vi "uc480_PixelPeek.vi"() -> ()   [LabVIEW 2011]
uses:
  C:/Program Files/Thorlabs/Scientific Imaging/DCx Camera Support/Develop/DotNet/uc480DotNet.dll
  Develop/DotNet/uc480DotNet.dll
panel:
  out "Maus":T1
  out "Blue":i32
  out "Green":i32
  out "Red":i32
  out "X":i32
  out "Y":i32
  out "Image":picture
  in  "Camera ID":i32 min=0 max=255
  out "Serial Number":string
  out "AOI Height":i32=8
  out "AOI Width":i32=8
  out "Bits/Pixel":i32=8
  out "Error Out":errorcluster caption="error"
  in  "Exit Camera":bool
  in  "Init Camera":bool
  # "Coordinates"
  # "Pixel Values"
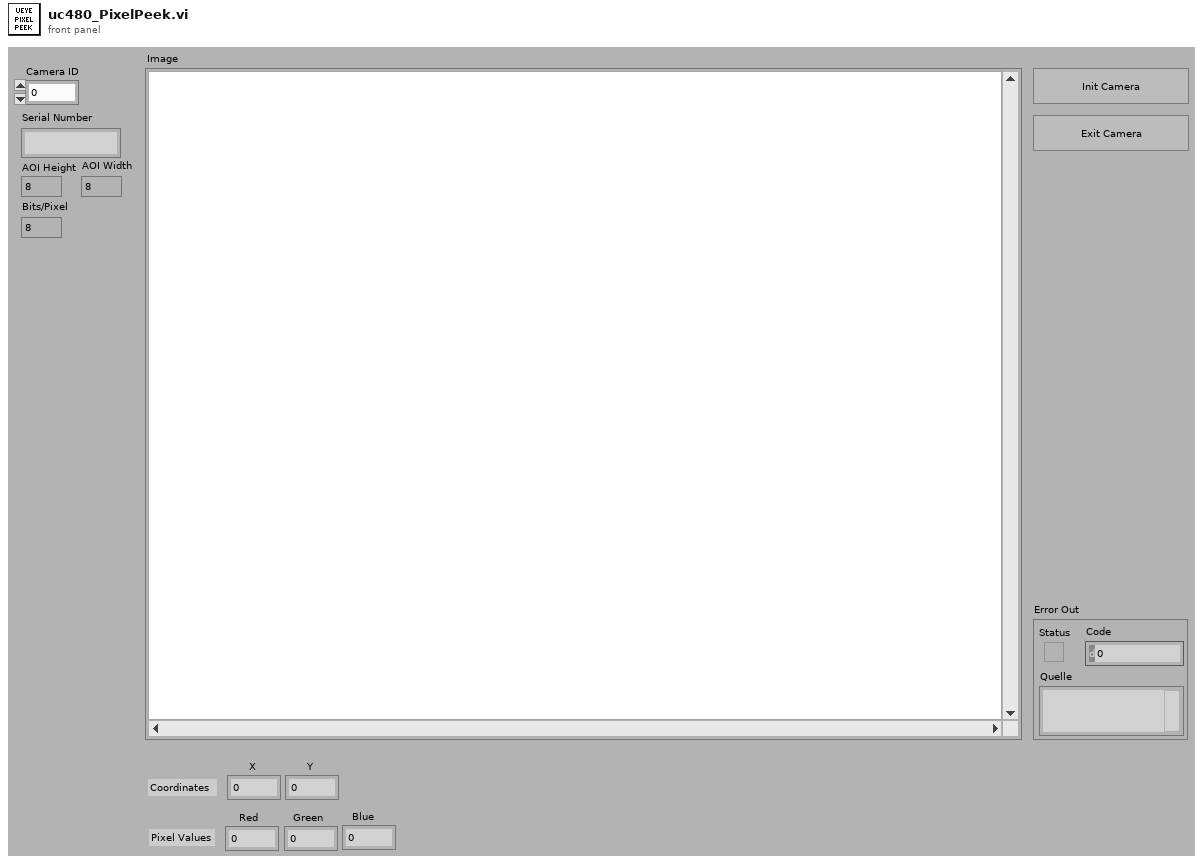
[diagram p1: front panel]
types:
  T1 = cluster{"Mouse Position":cluster{"X":i32, "Y":i32}, "Mouse Modifiers":cluster{"Button Down":bool, "Shift Mod":bool, "Menu Mod":bool, "Option Mod":bool}}
  T2 = enum8{"Enabled", "Disabled", "Disabled and Grayed Out"}
  T3 = typedef "LVMouseTypeDef.ctl" = cluster{"Mouse Position":cluster{"X":i32, "Y":i32}, "Mouse Modifiers":cluster{"Button Down":bool, "Shift Mod":bool, "Menu Mod":bool, "Option Mod":bool}}
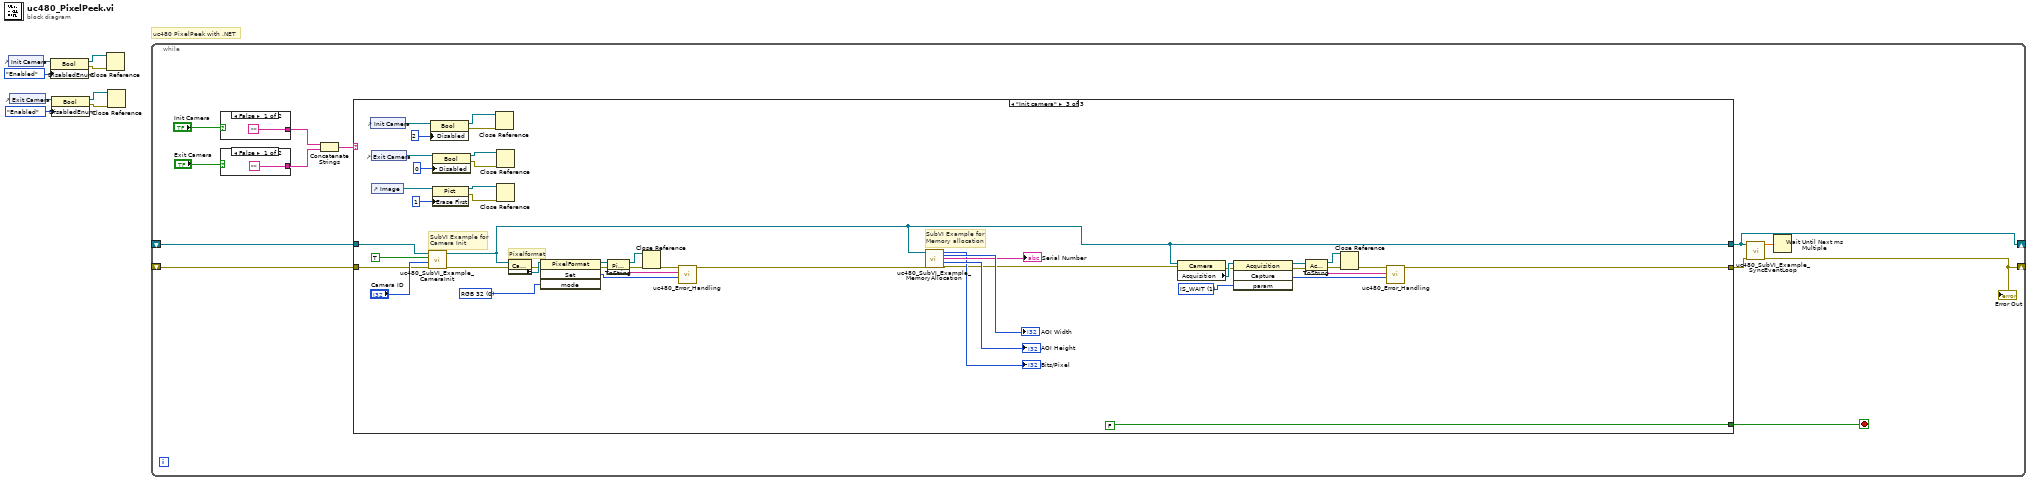
[diagram p0: block diagram]
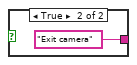
[diagram p2: hidden frame]
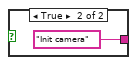
[diagram p3: hidden frame]
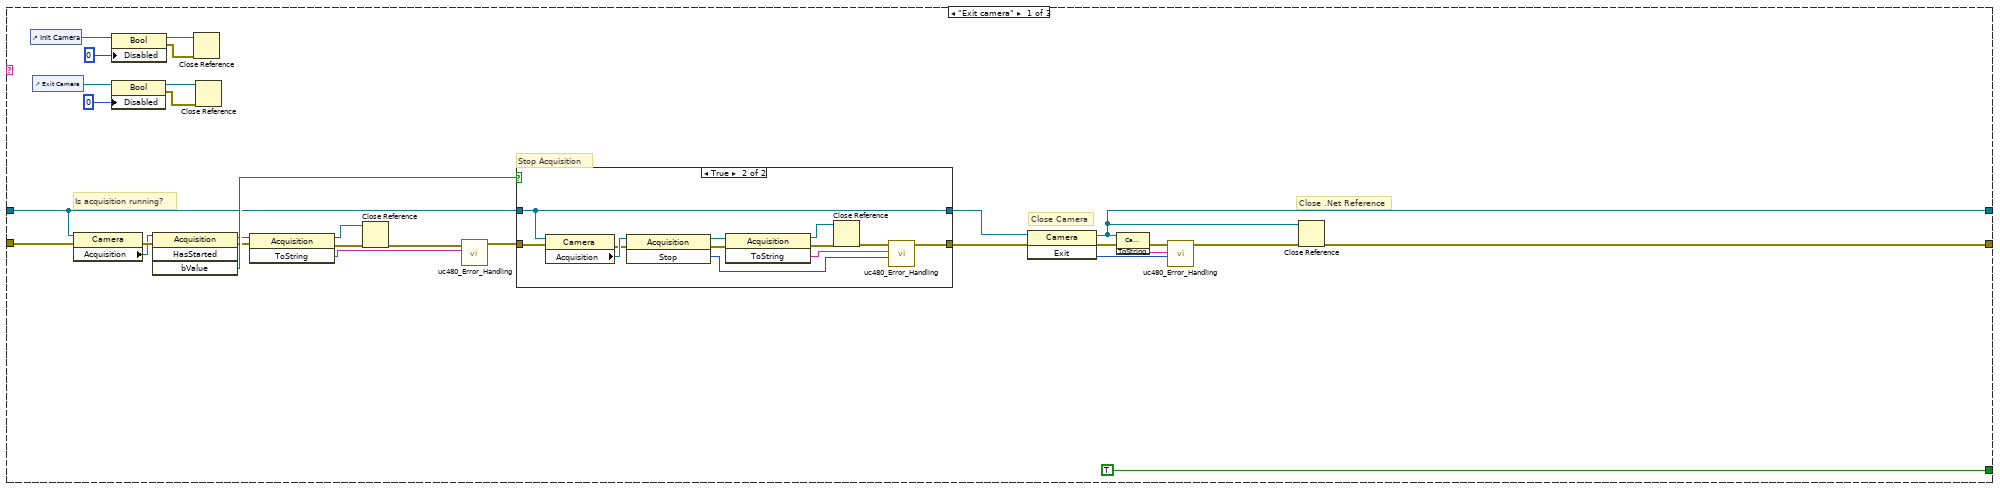
[diagram p4: hidden frame]
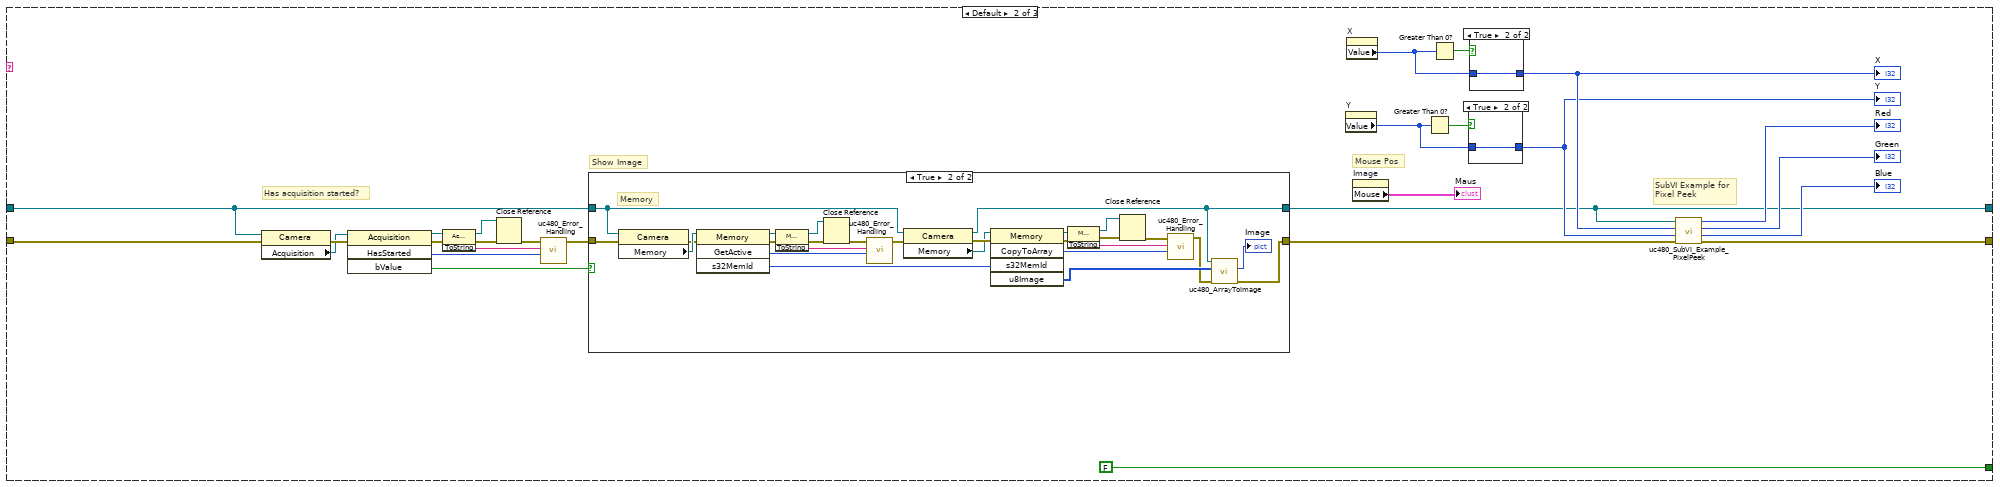
[diagram p6: hidden frame]
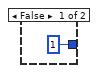
[diagram p7: hidden frame]
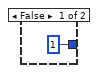
[diagram p8: hidden frame]
diagram:
  # "uc480 PixelPeek with .NET"
  n1 = control-ref of="Init Camera"() -> (w7:refnum<vi>)
  n2 = control-ref of="Exit Camera"() -> (w5:refnum<vi>)
  n3 = property class="Bool"(reference=w7, "DisabledEnum"=T2."Enabled" ("Disabled")) -> (reference out=w3:refnum<vi>, error out=w4:errorcluster)  [unwired: 1 in]
  n4 = property class="Bool"(reference=w5, "DisabledEnum"=T2."Enabled" ("Disabled")) -> (reference out=w2:refnum<vi>, error out=w1:errorcluster)  [unwired: 1 in]
  n5 = Close Reference ("Close Referenz")(reference=w3, error in (no error)=w4) -> ()  [unwired: 1 out]
  n6 = Close Reference ("Close Referenz")(reference=w2, error in (no error)=w1) -> ()  [unwired: 1 out]
  n7 = while {
    shift-right: [w12] -> _
    shift-left: _ -> [w15]
    shift-right: [w10] -> _
    shift-left: _ -> [w9]
    stop <- w14 stop-if-true
    n8 = case shown="False" "Exit Camera" {
      tunnel: ["" "Exit camera"] -> w16
      frame False {
      }
      frame True {
      }
    }
    n9 = case shown="False" "Init Camera" {
      tunnel: ["" "Init camera"] -> w19
      frame False {
      }
      frame True {
      }
    }
    n10 = Concatenate Strings(w19, w16) -> (w18:string)
    n11 = case shown="\"Init camera\"" w18 {
      tunnel: w9 -> [w38 w87 w166]
      tunnel: w15 -> [w39 w75 w165]
      tunnel: [w47 w74 w142] -> w10
      tunnel: [w48 w73 w150] -> w13
      tunnel: [TRUE FALSE FALSE] -> w14
      frame "Exit camera" {
        # "Close .Net Reference"
        # "Is acquisition running?"
        # "Stop Acquisition"
        # "Close Camera"
        n12 = control-ref of="Init Camera"() -> (w33:refnum<vi>)
        n13 = control-ref of="Exit Camera"() -> (w32:refnum<vi>)
        n14 = property class="Camera"(reference=w38, error in=w39) -> (error out=w46:errorcluster, "Acquisition"=w45:refnum<k24>)  [unwired: 1 out]
        n15 = property class="Bool"(reference=w32, "Disabled"=u8 0 ("Deaktiviert")) -> (reference out=w26:refnum<vi>, error out=w25:errorcluster)  [unwired: 1 in]
        n16 = property class="Bool"(reference=w33, "Disabled"=u8 0 ("Deaktiviert")) -> (reference out=w28:refnum<vi>, error out=w27:errorcluster)  [unwired: 1 in]
        n17 = invoke class="Acquisition" method="HasStarted"(reference=w45, error in=w46) -> (reference out=w40:refnum<k24>, error out=w42:errorcluster, "bValue"=w44:bool)  [unwired: 2 in, 1 out]
        n18 = Close Reference ("Close Referenz")(reference=w28, error in (no error)=w27) -> ()  [unwired: 1 out]
        n19 = Close Reference ("Close Referenz")(reference=w26, error in (no error)=w25) -> ()  [unwired: 1 out]
        n20 = invoke class="Acquisition" method="ToString"(reference=w40, error in=w42) -> (reference out=w29:refnum<k24>, error out=w31:errorcluster, "ToString"=w41:string)  [unwired: 1 in]
        n21 = Close Reference(reference=w29, error in (no error)=w31) -> (error out=w30:errorcluster)
        n22 = call "uc480_Error_Handling.vi"("Error String"=w41, "Error In"=w30) -> ("Error Out"=w43:errorcluster)  [unwired: 9 in]
        n23 = case shown="True" w44 {
          tunnel: [w56 w67] -> w36
          tunnel: w43 -> [w56 w68]
          tunnel: w38 -> [w55 w60]
          tunnel: [w55 w60] -> w37
          frame False {
          }
          frame True {
            n24 = property class="Camera"(reference=w60, error in=w68) -> (error out=w64:errorcluster, "Acquisition"=w65:refnum<k24>)  [unwired: 1 out]
            n25 = invoke class="Acquisition" method="Stop"(reference=w65, error in=w64) -> (reference out=w62:refnum<k24>, error out=w63:errorcluster, "Stop"=w61:i32)  [unwired: 1 in]
            n26 = invoke class="Acquisition" method="ToString"(reference=w62, error in=w63) -> (reference out=w57:refnum<k24>, error out=w59:errorcluster, "ToString"=w66:string)  [unwired: 1 in]
            n27 = Close Reference(reference=w57, error in (no error)=w59) -> (error out=w58:errorcluster)
            n28 = call "uc480_Error_Handling.vi"("Error Code"=w61, "Error String"=w66, "Error In"=w58) -> ("Error Out"=w67:errorcluster)  [unwired: 8 in]
          }
        }
        n29 = invoke class="Camera" method="Exit"(reference=w37, error in=w36) -> (reference out=w47:refnum<k24>, error out=w51:errorcluster, "Exit"=w50:i32)  [unwired: 1 in]
        n30 = invoke class="Camera" method="ToString"(reference=w47, error in=w51) -> (error out=w52:errorcluster, "ToString"=w53:string)  [unwired: 1 in, 1 out]
        n31 = call "uc480_Error_Handling.vi"("Error Code"=w50, "Error String"=w53, "Error In"=w52) -> ("Error Out"=w49:errorcluster)  [unwired: 8 in]
        n32 = Close Reference ("Close Referenz")(reference=w47, error in (no error)=w49) -> (error out=w48:errorcluster)
      }
      frame Default {
        # "SubVI Example for\nPixel Peek"
        # "Mouse Pos"
        # "Has acquisition started?"
        # "Show Image"
        n33 = property class="Camera"(reference=w87, error in=w75) -> (error out=w95:errorcluster, "Acquisition"=w94:refnum<k24>)  [unwired: 1 out]
        n34 = invoke class="Acquisition" method="HasStarted"(reference=w94, error in=w95) -> (reference out=w91:refnum<k24>, error out=w90:errorcluster, "HasStarted"=w89:i32, "bValue"=w93:bool)  [unwired: 2 in]
        n35 = invoke class="Acquisition" method="ToString"(reference=w91, error in=w90) -> (reference out=w69:refnum<k24>, error out=w71:errorcluster, "ToString"=w92:string)  [unwired: 1 in]
        n36 = Close Reference(reference=w69, error in (no error)=w71) -> (error out=w70:errorcluster)
        n37 = call "uc480_Error_Handling.vi"("Error Code"=w89, "Error String"=w92, "Error In"=w70) -> ("Error Out"=w88:errorcluster)  [unwired: 8 in]
        n38 = case shown="True" w93 {
          tunnel: [w101 w113] -> w82
          tunnel: w88 -> [w101 w114]
          tunnel: w87 -> [w100 w110]
          tunnel: [w100 w105] -> w74
          frame False {
          }
          frame True {
            # "Memory"
            n39 = property class="Camera"(reference=w110, error in=w114) -> (error out=w116:errorcluster, "Memory"=w117:refnum<k24>)  [unwired: 1 out]
            n40 = invoke class="Memory" method="GetActive"(reference=w117, error in=w116) -> (reference out=w122:refnum<k24>, error out=w121:errorcluster, "GetActive"=w123:i32, "s32MemId"=w115:i32)  [unwired: 2 in]
            n41 = invoke class="Memory" method="ToString"(reference=w122, error in=w121) -> (reference out=w106:refnum<k24>, error out=w108:errorcluster, "ToString"=w120:string)  [unwired: 1 in]
            n42 = Close Reference(reference=w106, error in (no error)=w108) -> (error out=w107:errorcluster)
            n43 = call "uc480_Error_Handling.vi"("Error Code"=w123, "Error String"=w120, "Error In"=w107) -> ("Error Out"=w124:errorcluster)  [unwired: 8 in]
            n44 = property class="Camera"(reference=w110, error in=w124) -> (reference out=w105:refnum<k24>, error out=w119:errorcluster, "Memory"=w118:refnum<k24>)
            n45 = invoke class="Memory" method="CopyToArray"(reference=w118, error in=w119, "s32MemId"=w115) -> (reference out=w126:refnum<k24>, error out=w127:errorcluster, "CopyToArray"=w128:i32, "u8Image"=w111:u8[])  [unwired: 2 in, 1 out]
            n46 = invoke class="Memory" method="ToString"(reference=w126, error in=w127) -> (reference out=w102:refnum<k24>, error out=w104:errorcluster, "ToString"=w125:string)  [unwired: 1 in]
            n47 = Close Reference(reference=w102, error in (no error)=w104) -> (error out=w103:errorcluster)
            n48 = call "uc480_Error_Handling.vi"("Error Code"=w128, "Error String"=w125, "Error In"=w103) -> ("Error Out"=w109:errorcluster)  [unwired: 8 in]
            n49 = call "uc480_ArrayToImage.vi"("Error In"=w109, "InArray"=w111, ".NET (Reference)"=w105) -> ("Error Out"=w113:errorcluster, "Image"=→"Image":picture)  [unwired: 7 in]
          }
        }
        n50 = property on="Y" class="DigNum (strict)"() -> ("Value"=w76:i32)  [unwired: 2 in, 2 out]
        n51 = property on="X" class="DigNum (strict)"() -> ("Value"=w77:i32)  [unwired: 2 in, 2 out]
        n52 = property on="Image" class="Pict"() -> ("Mouse"=→"Maus":T3)  [unwired: 2 in, 2 out]
        n53 = Greater Than 0?(x=w76) -> (x > 0?=w79:bool)
        n54 = Greater Than 0?(x=w77) -> (x > 0?=w78:bool)
        n55 = case shown="True" w79 {
          tunnel: w76 -> [_ w97]
          tunnel: [1 ("Value") w97] -> w80
          frame False {
          }
          frame True {
          }
        }
        "Y" <- w80
        n56 = case shown="True" w78 {
          tunnel: w77 -> [_ w99]
          tunnel: [1 ("Value") w99] -> w81
          frame False {
          }
          frame True {
          }
        }
        "X" <- w81
        n57 = call "uc480_SubVI_Example_PixelPeek.vi"("Error In"=w82, "Pos Y"=w80, "Pos X"=w81, ".NET (Reference)"=w74) -> ("Error Out"=w73:errorcluster, "Blue"=→"Blue":i32, "Green"=→"Green":i32, "Red"=→"Red":i32)  [unwired: 4 in]
      }
      frame "Init camera" {
        w151 = 1 items=["IS_DONT_WAIT", "IS_WAIT"] ("Wait")
        w174 = 0 items=["RGB 32"=0, "RGB 24"=1, "Y8 Monochrom"=6] ("Mode")
        # "SubVI Example for \nMemory allocation"
        # "SubVI Example for \nCamera Init"
        # "Pixelformat"
        n58 = control-ref of="Init Camera"() -> (w147:refnum<vi>)
        n59 = control-ref of="Exit Camera"() -> (w145:refnum<vi>)
        n60 = control-ref of="Image"() -> (w144:refnum<vi>)
        n61 = call "uc480_SubVI_Example_CameraInit.vi"("Error In"=w165, "Camera ID"="Camera ID", "Init Camera Flag"=TRUE, ".NET (Reference)"=w166) -> ("Error Out"=w171:errorcluster, ".NET (Reference)"=w142:refnum<k24>)  [unwired: 6 in]
        n62 = property class="Bool"(reference=w147, "Disabled"=u8 2 ("Deaktiviert")) -> (reference out=w132:refnum<vi>, error out=w131:errorcluster)  [unwired: 1 in]
        n63 = property class="Bool"(reference=w145, "Disabled"=u8 0 ("Deaktiviert")) -> (reference out=w133:refnum<vi>, error out=w130:errorcluster)  [unwired: 1 in]
        n64 = property class="Pict"(reference=w144, "Erase First"=u8 1) -> (reference out=w134:refnum<vi>, error out=w129:errorcluster)  [unwired: 1 in]
        n65 = Close Reference ("Close Referenz")(reference=w132, error in (no error)=w131) -> ()  [unwired: 1 out]
        n66 = Close Reference ("Close Referenz")(reference=w133, error in (no error)=w130) -> ()  [unwired: 1 out]
        n67 = Close Reference ("Close Referenz")(reference=w134, error in (no error)=w129) -> ()  [unwired: 1 out]
        n68 = property class="Camera"(reference=w142, error in=w171) -> (error out=w172:errorcluster, "PixelFormat"=w173:refnum<k24>)  [unwired: 1 out]
        n69 = invoke class="PixelFormat" method="Set"(reference=w173, error in=w172, "mode"=w174) -> (reference out=w169:refnum<k24>, error out=w162:errorcluster, "Set"=w168:i32)  [unwired: 1 in, 1 out]
        n70 = invoke class="PixelFormat" method="ToString"(reference=w169, error in=w162) -> (reference out=w138:refnum<k24>, error out=w140:errorcluster, "ToString"=w170:string)  [unwired: 1 in]
        n71 = Close Reference(reference=w138, error in (no error)=w140) -> (error out=w139:errorcluster)
        n72 = call "uc480_Error_Handling.vi"("Error Code"=w168, "Error String"=w170, "Error In"=w139) -> ("Error Out"=w141:errorcluster)  [unwired: 8 in]
        n73 = call "uc480_SubVI_Example_MemoryAllocation.vi"(".NET (Reference)"=w142, "Error In"=w141) -> ("Bits/Pixel 2"=→"Bits/Pixel":i32, "Width"=→"AOI Width":i32, "Serial Number"=→"Serial Number":string, "Height"=→"AOI Height":i32, "Error Out"=w149:errorcluster)  [unwired: 13 in]
        n74 = property class="Camera"(reference=w142, error in=w149) -> (error out=w156:errorcluster, "Acquisition"=w157:refnum<k24>)  [unwired: 1 out]
        n75 = invoke class="Acquisition" method="Capture"(reference=w157, error in=w156, "param"=w151) -> (reference out=w153:refnum<k24>, error out=w154:errorcluster, "Capture"=w152:i32)  [unwired: 1 in, 1 out]
        n76 = invoke class="Acquisition" method="ToString"(reference=w153, error in=w154) -> (reference out=w137:refnum<k24>, error out=w136:errorcluster, "ToString"=w155:string)  [unwired: 1 in]
        n77 = Close Reference(reference=w137, error in (no error)=w136) -> (error out=w135:errorcluster)
        n78 = call "uc480_Error_Handling.vi"("Error Code"=w152, "Error String"=w155, "Error In"=w135) -> ("Error Out"=w150:errorcluster)  [unwired: 8 in]
      }
    }
    n79 = call "uc480_SubVI_Example_SyncEventLoop.vi"("Error In"=w13, ".NET (Reference)"=w10) -> ("Error Out"=w12:errorcluster, "Synchronize (ms)"=w11:dbl)  [unwired: 8 in]
    "Error Out" <- w12
    n80 = Wait Until Next ms Multiple(millisecond multiple=w11) -> ()  [unwired: 1 out]
  }
